vi "Load TDMS Hierarchy.vi"(0 "Parent Ref in":T2 format="%.0x", 2 "interpolation settings":T1, 7 "file path":path, 11 "error in (no error)":errorcluster) -> (6 "dt out":dbl, 8 "Samples":u32, 15 "error out":errorcluster)   [LabVIEW 2011, in "TDMS Custom Device.lvlib"]
uses:
  TDMS Custom Device.lvlib
  <vilib>/NI Veristand/Custom Device API/Custom Device Item Ref.ctl
  <vilib>/NI Veristand/Custom Device API/Custom Device Channel.ctl
  <vilib>/NI Veristand/Custom Device API/Custom Device Channel Type.ctl
  <vilib>/NI Veristand/Custom Device API/Custom Device API.lvlib
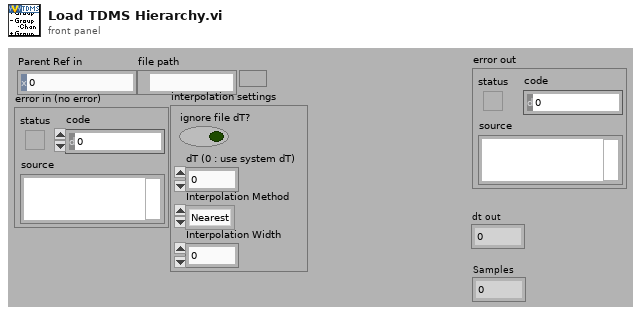
[diagram p1: front panel]
types:
  T1 = cluster{"ignore file dT?":bool, "dT (0 : use system dT)":dbl, "Interpolation Method ":enum16{"Nearest", "Linear", "Spline", "Cubic Hermite", "Lagrange", "Polynomial"}, "Interpolation Width":i32}
  T2 = typedef "Custom Device API.lvlib/Custom Device Item Ref.ctl" = u64
  T3 = enum16{"open", "open or create", "create or replace", "create", "open (read-only)"}
  T4 = typedef "Custom Device API.lvlib/Custom Device Channel.ctl" = cluster{"Type":T5, "Units":string, "Default Value":dbl, "Faultable":bool, "Scalable":bool}
  T5 = typedef "Custom Device API.lvlib/Custom Device Channel Type.ctl" = enum16{"Input", "Output"}
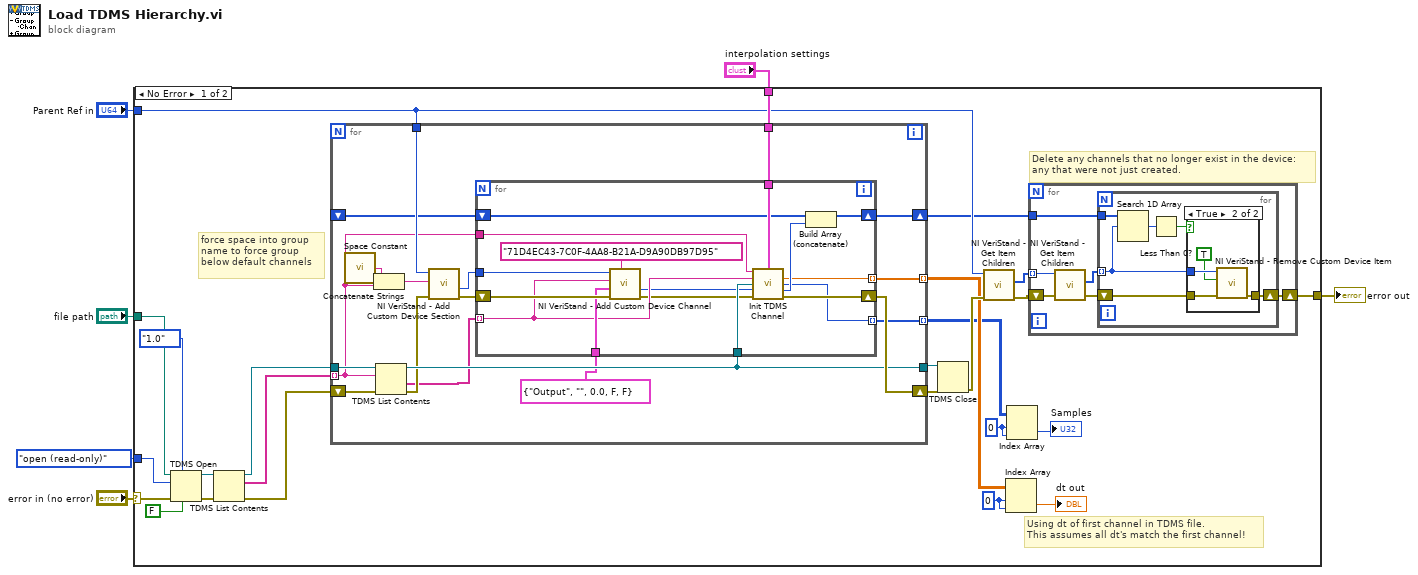
[diagram p0: block diagram]
diagram:
  n1 = case shown="No Error" "error in (no error)" {
    selector: "error in (no error)" -> [w25 w83]
    tunnel: T3."open (read-only)" ("operation (0:open)") -> [w31 _]
    tunnel: "Parent Ref in" -> [w23 _]
    tunnel: "file path" -> [w26 _]
    tunnel: [w18 w83] -> w3
    tunnel: "interpolation settings" -> [w24 _]
    frame No Error {
      w8 = 0 ("index (row)")
      w9 = 0 ("index (row)")
      # "force space into group\nname to force group \nbelow default channels"
      # "Using dt of first channel in TDMS file.\nThis assumes all dt's match the first channel!"
      # "Delete any channels that no longer exist in the device:\nany that were not just created."
      n2 = TDMS Open(6:FALSE ("disable buffering (T)"), 7:enum16{"1.0", "2.0"}."1.0" ("file format version (2.0)"), 8:w25, 10:w31, 11:w26) -> (0:w29:errorcluster, 3:w30:refnum<k34>)  [unwired: 1 in]
      n3 = TDMS List Contents(4:w29, 7:w30) -> (0:w27:errorcluster, 2:w11:string[], 3:w28:refnum<k34>)  [unwired: 2 out]
      n4 = for {
        tunnel: w11 -> [w51] mode=indexing
        tunnel: w28 -> [w66]
        shift-right: [w64] -> w20
        shift-left: w27 -> [w65]
        tunnel: [w63] -> w21
        tunnel: w23 -> [w62]
        tunnel: w24 -> [w61]
        shift-right: [w60] -> w16
        shift-left: _ -> [w59]
        tunnel: [w54] -> w13 mode=indexing
        tunnel: [w52] -> w10 mode=indexing
        n5 = call <vilib>:"Space Constant.vi"() -> ("String"=w49:string)
        n6 = Concatenate Strings(w49, w51) -> (w50:string)
        n7 = TDMS List Contents(4:w65, 6:w51, 7:w66) -> (0:w55:errorcluster, 1:w53:string[], 3:w63:refnum<k34>)  [unwired: 1 out]
        n8 = call <vilib>:"NI VeriStand - Add Custom Device Section.vi"("error in (no error)"=w55, "Section Name"=w50, "Parent Ref in"=w62) -> ("error out"=w58:errorcluster, "Section Ptr"=w57:T2)  [unwired: 4 in, 3 out]
        n9 = for {
          shift-right: [w82] -> w64
          shift-left: w58 -> [w80]
          tunnel: w57 -> [w81]
          tunnel: w53 -> [w78] mode=indexing
          tunnel: T4 {"Type"=enum."Output", "Units"="", "Default Value"=0.0, "Faultable"=FALSE, "Scalable"=FALSE} ("Channel") -> [w79]
          tunnel: w63 -> [w77]
          tunnel: w51 -> [w76]
          tunnel: w61 -> [w75]
          shift-right: [w74] -> w60
          shift-left: w59 -> [w73]
          tunnel: [w68] -> w54 mode=indexing
          tunnel: [w67] -> w52 mode=indexing
          n10 = call <vilib>:"NI VeriStand - Add Custom Device Channel.vi"("GUID (Default Channel)"="71D4EC43-7C0F-4AA8-B21A-D9A90DB97D95", "error in (no error)"=w80, "Channel"=w79, "Channel Name"=w78, "Parent Ref in"=w81) -> ("error out"=w72:errorcluster, "Channel Ref"=w70:T2)  [unwired: 3 in, 2 out]
          n11 = call "Init TDMS Channel.vi"("Group"=w76, "Interpolation Settings"=w75, "Channel"=w78, "tdms file"=w77, "Ref in"=w70, "error in (no error)"=w72) -> ("dt out"=w68:dbl, "Samples"=w67:u32, "Ref out"=w69:T2, "error out"=w82:errorcluster)  [unwired: 6 out]
          n12 = Build Array (concatenate)(w73, w69) -> (w74:T2[])
        }
      }
      n13 = TDMS Close(8:w20, 11:w21) -> (0:w19:errorcluster)  [unwired: 1 out]
      n14 = call <vilib>:"NI VeriStand - Get Item Children.vi"("error in (no error)"=w19, "Item Ref in"=w23) -> ("error out"=w22:errorcluster, "Child Refs"=w17:T2[])  [unwired: 8 out]
      n15 = Index Array(array=w13, index (row)=w9, index (col)=w9) -> (element=→"dt out":dbl)
      n16 = Index Array(array=w10, index (row)=w8, index (col)=w8) -> (element=→"Samples":u32)
      n17 = for {
        shift-right: [w36] -> w18
        shift-left: w22 -> [w37]
        tunnel: w17 -> [w34] mode=indexing
        tunnel: w16 -> [w32]
        n18 = call <vilib>:"NI VeriStand - Get Item Children.vi"("error in (no error)"=w37, "Item Ref in"=w34) -> ("error out"=w35:errorcluster, "Child Refs"=w33:T2[])  [unwired: 8 out]
        n19 = for {
          tunnel: w33 -> [w38] mode=indexing
          shift-right: [w43] -> w36
          shift-left: w35 -> [w42]
          tunnel: w32 -> [w41]
          n20 = Search 1D Array(1D array=w41, element=w38) -> (index of element=w39:i32)  [unwired: 1 out]
          n21 = Less Than 0?(x=w39) -> (x < 0?=w40:bool)
          n22 = case shown="True" w40 {
            tunnel: [w44 w48] -> w43
            tunnel: w42 -> [w44 w47]
            tunnel: w38 -> [_ w46]
            frame False {
            }
            frame True {
              n23 = call <vilib>:"NI VeriStand - Remove Custom Device Item.vi"("error in (no error)"=w47, "Force Delete (F)"=TRUE, "Item Ref in"=w46) -> ("error out"=w48:errorcluster)  [unwired: 8 out]
            }
          }
        }
      }
    }
    frame Error {
    }
  }
  "error out" <- w3
